vi "Image_Detect_Object_HQ.vi"(0 "Data":T3={"system"={"info"={"menuSelect"=0, "version"=0, "serial"="Test Sample", "captureActive"=FALSE, "captureBegin"=FALSE, "emptyAndRefill"=FALSE}, "userInfo"={"operatorName"="", "date"=timestamp(2713993200 s since 1904-01-01)}, "camera"={"exposureTime"=0, "aperture"=enum."Item 0", "framerate"=0, "framerateMax"=500, "legacyAttributes"=FALSE}}, "connections"={"arduino"={"connection"="MRJ", "status"=FALSE, "openState"=FALSE, "emptyStart"=0}, "pump"={"connection"="MRJ", "status"=FALSE, "command"="", "dispenseSpeed"=100, "flushSize"=100}, "camera"={"cam1"={"connection"="", "status"=FALSE}, "cam2"={"connection"="", "status"=FALSE}}}, "queue"={"process"={"cam1"=refnum, "cam2"=refnum, "queueSize"=0}, "save"={"cam1"=refnum, "cam2"=refnum, "queueSize"=0}, "overloadThreshold"=0}, "imageProcess"={"cam1"={"preAllocation"={"image"="Station", "originalDisplay"="Station", "originalRgb"="Station", "binary"="Station", "save"="Station", "calibrationFull"=refnum, "calibrationDetect"=refnum}, "calibration"={"pathFull"=path "C:/Users/au540322/Desktop/IHS_Project/images/Debris/Debris_0/Debris_0_2019_06_01-23-32-49-686.PNG", "pathDetect"=path "C:/Users/au540322/Desktop/IHS_Project/images/Debris/Debris_0/Debris_0_2019_06_01-23-32-49-686.PNG", "ROI"={"Left"=0, "Top"=0, "Right"=0, "Bottom"=0, "Rotation"=0.0}}}, "cam2"={"preAllocation"={"image"=refnum, "originalDisplay"=refnum, "originalRgb"=refnum, "binary"=refnum, "save"=refnum, "calibrationFull"=refnum, "calibrationDetect"=refnum}, "calibration"={"pathFull"=path "C:/Users/au540322/Desktop/IHS_Project/images/Debris/Debris_0/Debris_0_2019_06_01-23-32-49-686.PNG", "pathDetect"=path "C:/Users/au540322/Desktop/IHS_Project/images/Debris/Debris_0/Debris_0_2019_06_01-23-32-49-686.PNG", "ROI"={"Left"=0, "Top"=0, "Right"=0, "Bottom"=0, "Rotation"=0.0}}}, "process"={"planeExtract"=refnum, "planeSubtract"=refnum, "cropMask"=refnum}, "detection"={"sampleTimeout"=500, "sizeThreshold"=500, "detectionRegionPct"=0.0}}, "sampleData"={"sampleId"="", "projectId"="", "voucherID"="", "speciesName"="", "collectionDate"=timestamp(2713993200 s since 1904-01-01), "sampleStation"="", "location"="", "lat"=0.0, "lon"=0.0, "determiner"="", "sex"="", "otherNotes"=""}, "Session In"=""} {"sampleData"."collectionDate" format="%<%Y-%m-%d>T"; "imageProcess"."detection"."sizeThreshold" min=1; "imageProcess"."cam2"."calibration"."ROI"."Rotation" format="%.2f"; "imageProcess"."cam2"."calibration"."ROI"."Left" scale=0.0..1024.0; "imageProcess"."cam2"."calibration"."ROI"."Right" scale=0.0..1024.0; "imageProcess"."cam1"."calibration"."ROI"."Rotation" format="%.2f"; "imageProcess"."cam1"."calibration"."ROI"."Left" scale=0.0..1024.0; "imageProcess"."cam1"."calibration"."ROI"."Right" scale=0.0..1024.0; "queue"."overloadThreshold" min=1; "queue"."save"."queueSize" min=1; "queue"."process"."queueSize" min=1; "connections"."pump"."flushSize" min=1; "connections"."pump"."dispenseSpeed" min=1; "system"."camera"."framerateMax" min=1; "system"."userInfo"."date" format="%<%Y-%m-%dT%H:%M:%S+%z>T"; "system"."info"."version" items=["Standard", "XL"]; "system"."info"."menuSelect" items=["Session Data", "Extended Setup", "Buffer", "Camera", "Dispenser", "Stats", "Connections"]}, 5 "Image Pixels (U32)":u32[][](array[numeric]), 9 "Detect Crop":bool, 12 "Camera":T6=enum."Camera 2") -> (2 "error out":errorcluster, 3 "Obj Size":bool, 4 "Detected object":T1, 6 "Image Out":T1, 8 "Binary":T1, 10 "Object Accept":bool, 14 "ROI descriptor":T2, 15 "Sample Data":dbl[](array[numeric]))   [LabVIEW 2022 SP3]
uses:
  Camera_ID.ctl
  controls/Data.ctl
  <vilib>/userdefined/High Color/IMAQdx.ctl
  <vilib>/vision/Image Controls.llb/IMAQ Image.ctl
  <vilib>/vision/NI_Vision_Development_Module.lvlib
panel:
  in  "error in":errorcluster
  in  "Threshold":cluster{"Lower value":sgl, "Upper value":sgl}={"Lower value"=15.0, "Upper value"=256.0} {"Upper value" format="%.2f"; "Lower value" format="%.2f"}
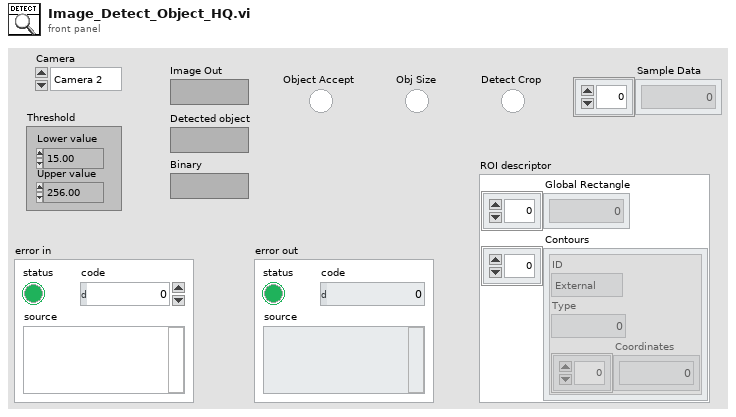
[diagram p1: front panel]
types:
  T1 = typedef "IMAQ Image.ctl" = refnum<image>
  T2 = cluster{"Global Rectangle":i32[], "Contours":cluster{"ID":enum32{"External", "Internal"}, "Type":u32, "Coordinates":i32[]}[]}
  T3 = typedef "Data.ctl" = cluster{"system":cluster{"info":cluster{"menuSelect":u16, "version":u16, "serial":string, "captureActive":bool, "captureBegin":bool, "emptyAndRefill":bool}, "userInfo":cluster{"operatorName":string, "date":timestamp}, "camera":cluster{"exposureTime":i32, "aperture":enum32{"Item 0", "Item 1", "Item 2", "Item 3"}, "framerate":i32, "framerateMax":i32, "legacyAttributes":bool}}, "connections":cluster{"arduino":cluster{"connection":refnum<visa-resource-name>, "status":bool, "openState":bool, "emptyStart":u32}, "pump":cluster{"connection":refnum<visa-resource-name>, "status":bool, "command":string, "dispenseSpeed":i32, "flushSize":i32}, "camera":cluster{"cam1":cluster{"connection":T4, "status":bool}, "cam2":cluster{"connection":T4, "status":bool}}}, "queue":cluster{"process":cluster{"cam1":refnum<queue>, "cam2":refnum<queue>, "queueSize":i32}, "save":cluster{"cam1":refnum<queue>, "cam2":refnum<queue>, "queueSize":i32}, "overloadThreshold":i32}, "imageProcess":cluster{"cam1":cluster{"preAllocation":cluster{"image":T1, "originalDisplay":T1, "originalRgb":T1, "binary":T1, "save":T1, "calibrationFull":T1, "calibrationDetect":T1}, "calibration":cluster{"pathFull":path, "pathDetect":path, "ROI":T5}}, "cam2":cluster{"preAllocation":cluster{"image":T1, "originalDisplay":T1, "originalRgb":T1, "binary":T1, "save":T1, "calibrationFull":T1, "calibrationDetect":T1}, "calibration":cluster{"pathFull":path, "pathDetect":path, "ROI":T5}}, "process":cluster{"planeExtract":T1, "planeSubtract":T1, "cropMask":T1}, "detection":cluster{"sampleTimeout":i32, "sizeThreshold":i32, "detectionRegionPct":dbl}}, "sampleData":cluster{"sampleId":string, "projectId":string, "voucherID":string, "speciesName":string, "collectionDate":timestamp, "sampleStation":string, "location":string, "lat":dbl, "lon":dbl, "determiner":string, "sex":string, "otherNotes":string}, "Session In":T4}
  T4 = typedef "IMAQdx.ctl" = refnum<k21>
  T5 = typedef "IMAQ Rectangle" = cluster{"Left":i32, "Top":i32, "Right":i32, "Bottom":i32, "Rotation":dbl}
  T6 = typedef "Camera_ID.ctl" = enum16{"Camera 1", "Camera 2"}
  T7 = typedef "Particle Parameters" = i32
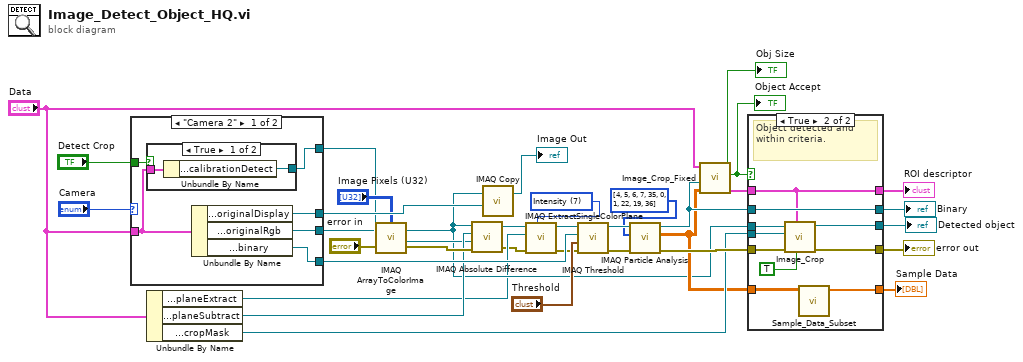
[diagram p0: block diagram]
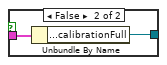
[diagram p2: hidden frame]
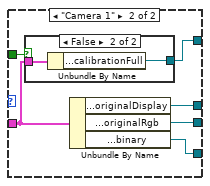
[diagram p3: hidden frame]
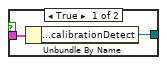
[diagram p4: hidden frame]
diagram:
  w10 = 7 items=["Red", "Green", "Blue", "Hue", "Saturation", "Luminance", "Value", "Intensity"] ("Color Plane")
  w20 = T7[] [4, 5, 6, 7, 35, 0, 1, 22, 19, 36] items=["Center of Mass X", "Center of Mass Y", "First Pixel X", "First Pixel Y", "Bounding Rect Left", "Bounding Rect Top", "Bounding Rect Right", "Bounding Rect Bottom", "Max Feret Diameter Start X", "Max Feret Diameter Start Y", "Max Feret Diameter End X", "Max Feret Diameter End Y", "Max Horiz. Segment Length Left", "Max Horiz. Segment Length Right", "Max Horiz. Segment Length Row", "-", "Bounding Rect Width", "Bounding Rect Height", "Bounding Rect Diagonal", "Perimeter", "Convex Hull Perimeter", "Holes' Perimeter", "Max Feret Diameter", "Equivalent Ellipse Major Axis", "Equivalent Ellipse Minor Axis", "Equivalent Ellipse Minor Axis (Feret)", "Equivalent Rect Long Side", "Equivalent Rect Short Side", "Equivalent Rect Diagonal", "Equivalent Rect Short Side (Feret)", "Average Horiz. Segment Length", "Average Vert. Segment Length", "Hydraulic Radius", "Waddel Disk Diameter", "-", "Area", "Holes' Area", "Particle & Holes' Area", "Convex Hull Area", "Image Area", "-", "Number of Holes", "Number of Horiz. Segments", "Number of Vert. Segments", "-", "Orientation", "Max Feret Diameter Orientation", "-", "% Area/Image Area", "% Area/(Particle & Holes' Area)", "Ratio of Equivalent Ellipse Axes", "Ratio of Equivalent Rect Sides", "-", "Elongation Factor", "Compactness Factor", "Heywood Circularity Factor", "Type Factor", "-", "Sum X", "Sum Y", "Sum XX", "Sum XY", "Sum YY", "Sum XXX", "Sum XXY", "Sum XYY", "Sum YYY", "-", "Moment of Inertia XX", "Moment of Inertia XY", "Moment of Inertia YY", "Moment of Inertia XXX", "Moment of Inertia XXY", "Moment of Inertia XYY", "Moment of Inertia YYY", "Norm. Moment of Inertia XX", "Norm. Moment of Inertia XY", "Norm. Moment of Inertia YY", "Norm. Moment of Inertia XXX", "Norm. Moment of Inertia XXY", "Norm. Moment of Inertia XYY", "Norm. Moment of Inertia YYY", "Hu Moment 1", "Hu Moment 2", "Hu Moment 3", "Hu Moment 4", "Hu Moment 5", "Hu Moment 6", "Hu Moment 7"] ("Pixel Measurements")
  n1 = case shown="\"Camera 2\"" "Camera" {
    tunnel: "Data" -> [w40 w50]
    tunnel: [w39 w49] -> w12
    tunnel: [w37 w48] -> w9
    tunnel: [w38 w46] -> w26
    tunnel: "Detect Crop" -> [w41 w51]
    tunnel: [w36 w47] -> w18
    frame "Camera 2" {
      n2 = case shown="True" w41 {
        tunnel: w40 -> [w43 w45]
        tunnel: [w42 w44] -> w39
        frame True {
          n3 = Unbundle By Name(w43) -> ("imageProcess.cam2.preAllocation.calibrationDetect"=w42:T1)
        }
        frame False {
          n4 = Unbundle By Name(w45) -> ("imageProcess.cam2.preAllocation.calibrationFull"=w44:T1)
        }
      }
      n5 = Unbundle By Name(w40) -> ("imageProcess.cam2.preAllocation.originalDisplay"=w36:T1, "imageProcess.cam2.preAllocation.originalRgb"=w37:T1, "imageProcess.cam2.preAllocation.binary"=w38:T1)
    }
    frame "Camera 1" {
      n6 = case shown="False" w51 {
        tunnel: w50 -> [w53 w55]
        tunnel: [w52 w54] -> w49
        frame True {
          n7 = Unbundle By Name(w53) -> ("imageProcess.cam1.preAllocation.calibrationDetect"=w52:T1)
        }
        frame False {
          n8 = Unbundle By Name(w55) -> ("imageProcess.cam1.preAllocation.calibrationFull"=w54:T1)
        }
      }
      n9 = Unbundle By Name(w50) -> ("imageProcess.cam1.preAllocation.originalDisplay"=w47:T1, "imageProcess.cam1.preAllocation.originalRgb"=w48:T1, "imageProcess.cam1.preAllocation.binary"=w46:T1)
    }
  }
  n10 = Unbundle By Name("Data") -> ("imageProcess.process.planeExtract"=w7:T1, "imageProcess.process.planeSubtract"=w13:T1, "imageProcess.process.cropMask"=w27:T1)
  n11 = call "IMAQ ArrayToColorImage"("Image Pixels (U32)"="Image Pixels (U32)", "Image"=w9, "error in (no error)"="error in") -> ("Image Out"=w8:T1, "error out"=w15:errorcluster)  [unwired: 2 in]
  n12 = call "IMAQ Absolute Difference"("Image Src A"=w8, "Image Dst"=w13, "Image Src B"=w12, "error in (no error)"=w15) -> ("Image Dst Out"=w11:T1, "error out"=w5:errorcluster)  [unwired: 3 in]
  n13 = call "IMAQ Copy"("Image Dst"=w18, "Image Src"=w8) -> ("Image Dst Out"=→"Image Out":T1)  [unwired: 4 in, 1 out]
  n14 = call "IMAQ ExtractSingleColorPlane"("Color Plane"=w10, "error in (no error)"=w5, "Image Dst"=w7, "Image Src"=w11) -> ("error out"=w4:errorcluster, "Image Dst Out"=w6:T1)  [unwired: 6 out]
  n15 = call "IMAQ Threshold"("error in (no error)"=w4, "Range"="Threshold", "Image Dst"=w26, "Image Src"=w6) -> ("error out"=w30:errorcluster, "Image Dst Out"=w32:T1)  [unwired: 2 in, 4 out]
  n16 = call "IMAQ Particle Analysis"("error in (no error)"=w30, "Pixel Measurements"=w20, "Image"=w32) -> ("error out"=w33:errorcluster, "Particle Measurements (Pixels)"=w22:dbl[][], "Image Out (duplicate)"=w34:T1)  [unwired: 2 in, 4 out]
  n17 = call "Image_Crop_Fixed.vi"("Particle Measurements"=w22, "Image  in"=w34, "Data"="Data") -> ("ROI descriptor"=w35:T2, "Object accept"=w25:bool, "Object"=→"Obj Size":bool)  [unwired: 6 in]
  "Object Accept" <- w25
  n18 = case shown="True" w25 {
    tunnel: [w56 w67] -> w1
    tunnel: w33 -> [w57 w65]
    tunnel: [w58 w66] -> w2
    tunnel: w34 -> [w58 w66]
    tunnel: [w57 w64] -> w14
    tunnel: w35 -> [_ w60]
    tunnel: w27 -> [_ w59]
    tunnel: w8 -> [w56 w63]
    tunnel: w22 -> [_ w62]
    tunnel: [_ w61] -> w21
    tunnel: [_ w60] -> w16
    frame False {
      # "No object found or not within criteria."
    }
    frame True {
      # "Object detected and within criteria."
      n19 = call "Image_Crop.vi"("Shrink"=TRUE, "ROI Descriptor"=w60, "error in (no error)"=w65, "Image Dest"=w59, "Image Src"=w63) -> ("error out"=w64:errorcluster, "Image Out"=w67:T1)  [unwired: 5 in]
      n20 = call "Sample_Data_Subset.vi"("Particle Measurements (Pixels)"=w62) -> ("Sample Data"=w61:dbl[])  [unwired: 10 in]
    }
  }
  "error out" <- w14
  "Sample Data" <- w21
  "ROI descriptor" <- w16
  "Detected object" <- w1
  "Binary" <- w2
